vi "New Item.vi"(8 "error in (no error)":errorcluster, 10 "Item Configuration":T1, 11 "Assert Display in":refnum<class "Assert Display.lvclass">) -> (0 "error out":errorcluster, 3 "Assert Display out":refnum<class "Assert Display.lvclass">)   [LabVIEW 2016, in "Assert API Components.lvlib" / "Assert Display.lvlib" / "Assert Display.lvclass"]
uses:
  Assert Display.lvclass
  Item Configuration.ctl
  Service Config Display/Service Config Display/Items.ctl
  Assert Display.lvclass/Assert Display.ctl
  Service Config Display/Service Config Display/Service Details.ctl
  Main Display/Main Display Messages/Create UDP Service Msg/Create UDP Service Msg.lvclass/Create UDP Service Msg.ctl
  <vilib>/ActorFramework/Message Enqueuer/Message Enqueuer.lvclass/Message Enqueuer.ctl
  Assert API Components/Filter Configurations/Base Filter.lvclass
  Main Display/Main Display Messages/Configure Filter Msg/Configure Filter Msg.lvclass/Configure Filter Msg.ctl
  <vilib>/ActorFramework/Message Enqueuer/Enqueue.vi
  Main Display/Main Display Messages/Create UDP Service Msg/Create UDP Service Msg.lvclass
  C:/Program Files (x86)/National Instruments/LabVIEW 2016/vi.lib/ActorFramework/Message/Message.lvclass
  Main Display/Main Display Messages/Configure Filter Msg/Configure Filter Msg.lvclass
  <vilib>/Utility/LVClass/Get LV Class Name.vi
  <resource>/AFDebug/Generate Trace for Message.vi
  <vilib>/ActorFramework/Message Priority Queue/Priority Enqueue.vi
  Assert Display.lvlib
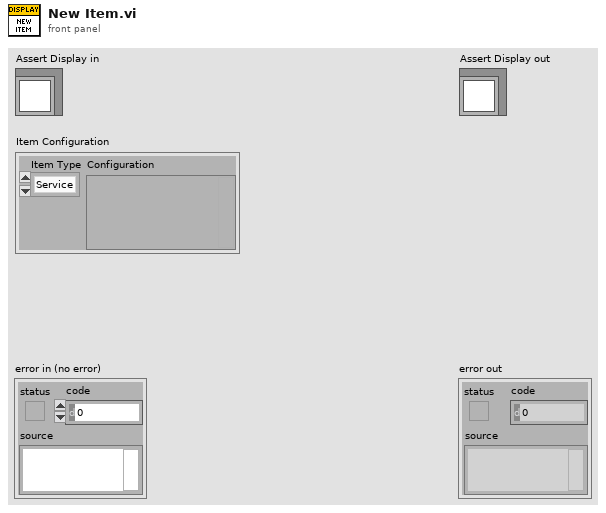
[diagram p1: front panel]
types:
  T1 = typedef "Assert API Components.lvlib/Assert Display.lvlib/Item Configuration.ctl" = cluster{"Item Type":T2, "Configuration":variant}
  T2 = typedef "Assert API Components.lvlib/Assert Display.lvlib/Items.ctl" = enum16{"Service", "Filter"}
  T3 = typedef "Assert API Components.lvlib/Assert Display.lvlib/Service Details.ctl" = cluster{"Name":string, "IP Address":string}
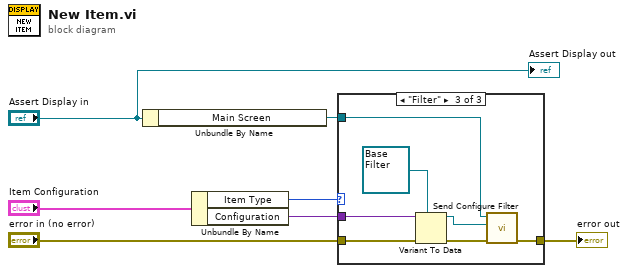
[diagram p0: block diagram]
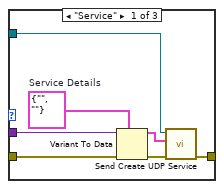
[diagram p2: hidden frame]
diagram:
  n1 = Unbundle By Name("Assert Display in") -> ("Main Screen"=w4:refnum<class "Message Enqueuer.lvclass">)
  n2 = Unbundle By Name("Item Configuration") -> ("Item Type"=w6:T2, "Configuration"=w5:variant)
  n3 = case shown="\"Filter\"" w6 {
    tunnel: w5 -> [w14 _ w19]
    tunnel: w4 -> [w11 _ w17]
    tunnel: "error in (no error)" -> [w12 w15 w22]
    tunnel: [w8 w15 w21] -> w1
    frame "Service" {
      w13 = T3 {"Name"="", "IP Address"=""}  # Service Details
      n4 = Variant To Data(error in=w12, type=w13, Variant=w14) -> (data=w10:T3, error out=w9:errorcluster)
      n5 = call "Send Create UDP Service.vi"("error in (no error)"=w9, "Service Details"=w10, "Message Enqueuer"=w11) -> ("error out"=w8:errorcluster)  [unwired: 7 in, 1 out]
    }
    frame Default {
    }
    frame "Filter" {
      n6 = Variant To Data(error in=w22, type=refnum<class "Base Filter.lvclass"> refnum ("New Filter"), Variant=w19) -> (data=w16:refnum<class "Base Filter.lvclass">, error out=w20:errorcluster)
      n7 = call "Send Configure Filter.vi"("error in (no error)"=w20, "New Filter"=w16, "Message Enqueuer"=w17) -> ("error out"=w21:errorcluster)  [unwired: 7 in, 1 out]
    }
  }
  "error out" <- w1
  "Assert Display out" <- "Assert Display in"
